vi "GetSettings.vi"(8 "error in (no error)":errorcluster, 10 "SettingsToRetrieve":variant, 11 "NHRGridSim in":refnum<class "NHRGridSim.lvclass">) -> (0 "error out":errorcluster, 1 "DeviceConfig&Meas":variant, 2 "RetrievedSettings":variant, 3 "NHRGridSim Out":refnum<class "NHRGridSim.lvclass">)   [LabVIEW 2018, in "AcPwrPlugins.lvlib" / "NHRGridSim.lvclass"]
doc: "This VI retrieves a boolean status to see if the instrument can conduct measurements while the device is changing modes or turning off and on."
uses:
  NHRGridSim.lvclass
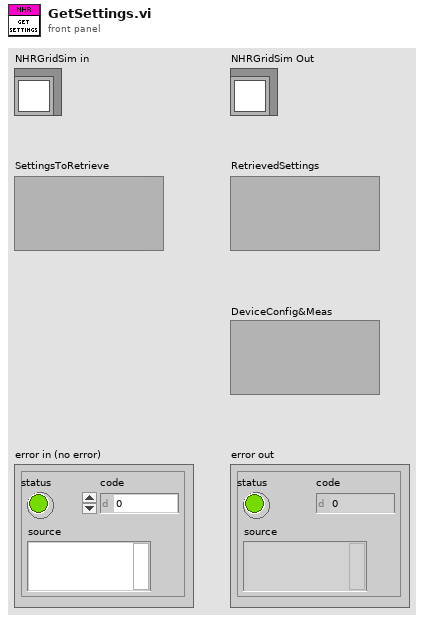
[diagram p1: front panel]
types:
  T1 = typedef "AcPwrPlugins.lvlib/NHRGridSim.lvclass/Device(s)Settings.ctl" = cluster{"MeasName":string, "Modules":T2}
  T2 = typedef "AcPwrPlugins.lvlib/NHRGridSim.lvclass/Modules.ctl" = cluster{"Measurement":cluster{"ApertureLength (s)":dbl, "NumberOfSamples":u32}, "Ranges":cluster{"Irange (A)":dbl, "Vrange (V)":dbl}, "Mode":u8, "Handle":string, "FreqOut (Hz)":dbl, "Connected":bool, "btnIdQuery":bool, "btnReset":bool, "Initialize Timeout ( ms)":u32, "Phase (0: All)":i32, "WatchDog":cluster{"Enable WatchDog":bool, "Robust WatchDog":bool, "Watchdog Interval (s)":dbl}, "Safety Limits":cluster{"Min Voltage (V)":dbl, "Min Voltage Time (s)":dbl, "Max Voltage (V)":dbl, "MaxVoltage Time (s)":dbl, "Max Source Amps (A)":dbl, "Max Source Amps Time (s)":dbl, "Max Sink Amps (A)":dbl, "Max Sink Amps Time (s)":dbl, "Max Source Power (W)":dbl, "Max Source Power Time (s)":dbl, "Max Sink Power (W)":dbl, "Max Sink Power Time (s)":dbl, "Peak Voltage (V)":dbl, "Peak Voltage Enable":bool, "Peak Amps (A)":dbl, "Peak Amps Enable":bool}, "Phases":cluster{"Pout (W)":dbl, "Iout (A)":dbl, "PhaseAngle":dbl, "Vout (V)":dbl, "Phase Name":string}[], "Regulation Gain":dbl, "ChangeOntheFly":bool, "Synchronize Output \nto Phase":bool, "Slew Rate":cluster{"Voltage Slew (Volts/s)":dbl, "Phase Angle (Degrees/s)":dbl}}[]
  T3 = typedef "AcPwrPlugins.lvlib/NHRGridSim.lvclass/Measurements.ctl" = cluster{"Handle":string, "Name":string, "Enabled ":bool, "Measurement Value":dbl, "Phase ":i32, "Measurement Type ":T4}[]
  T4 = typedef "AcPwrPlugins.lvlib/NHRGridSim.lvclass/MeasurementType.ctl" = enum16{"Average Current", "Average Voltage"}
  T5 = cluster{"xml string":string, "xml string":string}
  T6 = cluster{"Device(s)Settings":T1, "Measurements":T3}
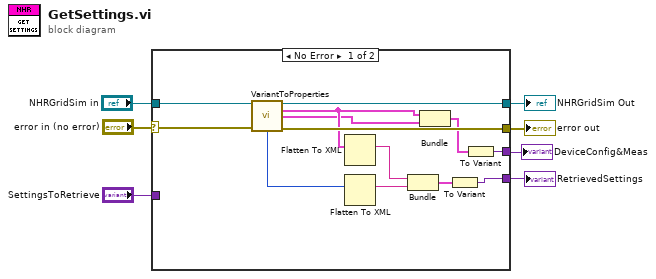
[diagram p0: block diagram]
diagram:
  n1 = case shown="No Error" "error in (no error)" {
    selector: "error in (no error)" -> [w19 w22]
    tunnel: "NHRGridSim in" -> [w20 w23]
    tunnel: [w18 w23] -> w6
    tunnel: [w17 w22] -> w2
    tunnel: "SettingsToRetrieve" -> [_ w21]
    tunnel: [w12 w21] -> w3
    tunnel: [w8 _] -> w1
    frame No Error {
      n2 = call "VariantToProperties.vi"("NHRGridSim in"=w20, "error in (no error)"=w19) -> ("NHRGridSim out"=w18:refnum<class "NHRGridSim.lvclass">, "Device(s)Settings"=w11:T1, "Measurements"=w10:T3, "Measurement Refresh Time (ms)"=w13:u32, "error out"=w17:errorcluster)  [unwired: 7 in, 2 out]
      n3 = Flatten To XML(anything=w11) -> (xml string=w15:string)
      n4 = Flatten To XML(anything=w13) -> (xml string=w14:string)
      n5 = Bundle("xml string"=w15, "xml string"=w14) -> (w16:T5)  [unwired: 1 in]
      n6 = Bundle("Device(s)Settings"=w11, "Measurements"=w10) -> (w9:T6)  [unwired: 1 in]
      n7 = To Variant(anything=w16) -> (Variant=w12:variant)
      n8 = To Variant(anything=w9) -> (Variant=w8:variant)
    }
    frame Error {
    }
  }
  "error out" <- w2
  "NHRGridSim Out" <- w6
  "RetrievedSettings" <- w3
  "DeviceConfig&Meas" <- w1
